vi "Pidadjus.vi"(1 "GPIB ADDRESS":string, 2 "RESET (Inetegral)":ext(knob) scale=0.1..99.0 scale format="%.1f", 3 "RATE (Derivative)":ext(knob) scale=0.1..99.0 scale format="%.1f", 4 "GAIN (Proportional)":ext(knob) scale=0.1..99.0 scale format="%.1f", 5 "?":bool) -> (0 "PID Return Testor":string)   [LabVIEW 2020]
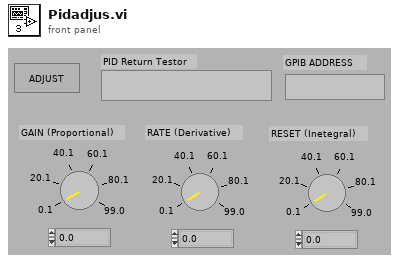
[diagram p1: front panel]
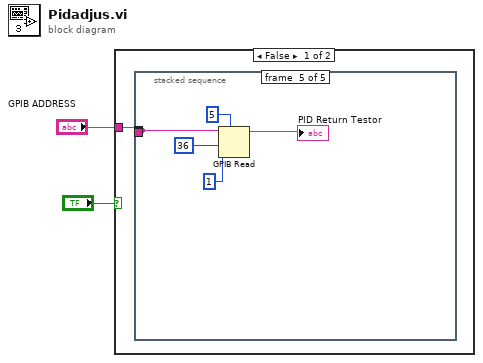
[diagram p0: block diagram]
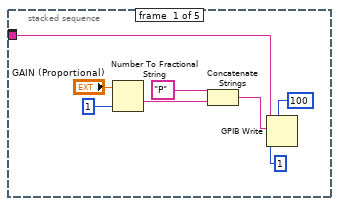
[diagram p2: hidden frame]
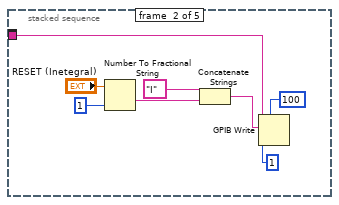
[diagram p3: hidden frame]
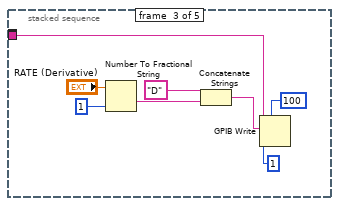
[diagram p4: hidden frame]
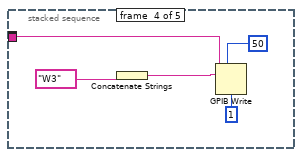
[diagram p5: hidden frame]
diagram:
  n1 = case shown="False" "?" {
    tunnel: "GPIB ADDRESS" -> [w3 _]
    frame False {
      n2 = stacked-sequence {
        tunnel: w3 -> [_ _ _ _ w33]
        tunnel: w3 -> [_ _ _ w32 _]
        tunnel: w3 -> [w4 w12 w21 _ _]
        frame #0 {
          n3 = Number To Fractional String(number="GAIN (Proportional)", precision (6)=1) -> (F-format string=w8:string)  [unwired: 2 in]
          n4 = Concatenate Strings("P", w8) -> (w5:string)
          n5 = GPIB Write(0:w4, 1:w5, 2:1, 4:100) -> ()  [unwired: 1 in, 2 out]
        }
        frame #1 {
          n6 = Number To Fractional String(number="RESET (Inetegral)", precision (6)=1) -> (F-format string=w16:string)  [unwired: 2 in]
          n7 = Concatenate Strings("I", w16) -> (w13:string)
          n8 = GPIB Write(0:w12, 1:w13, 2:1, 4:100) -> ()  [unwired: 1 in, 2 out]
        }
        frame #2 {
          n9 = Number To Fractional String(number="RATE (Derivative)", precision (6)=1) -> (F-format string=w20:string)  [unwired: 2 in]
          n10 = Concatenate Strings("D", w20) -> (w22:string)
          n11 = GPIB Write(0:w21, 1:w22, 2:1, 4:100) -> ()  [unwired: 1 in, 2 out]
        }
        frame #3 {
          n12 = Concatenate Strings("W3") -> (w29:string)
          n13 = GPIB Write(0:w32, 1:w29, 2:1, 4:50) -> ()  [unwired: 1 in, 2 out]
        }
        frame #4 {
          n14 = GPIB Read(0:w33, 1:36, 2:1, 4:5) -> (5:→"PID Return Testor":string)  [unwired: 1 in, 2 out]
        }
      }
    }
    frame True {
    }
  }
